vi "Calcula delay.vi"(8 "error in":errorcluster, 10 "ms in":u32) -> (0 "error out":errorcluster, 1 "delay":u32, 2 "ms out":u32)   [LabVIEW 2018]
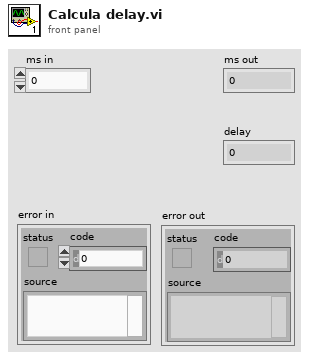
[diagram p1: front panel]
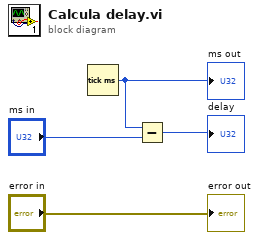
[diagram p0: block diagram]
diagram:
  n1 = Tick Count (ms)() -> (millisecond timer value=w4:u32)
  "ms out" <- w4
  n2 = Subtract(x=w4, y="ms in") -> (x-y=→"delay":u32)
  "error out" <- "error in"
